vi "Data.vi"(8 "error in (no error)":errorcluster, 11 "PB Msg Template in":refnum<class "Msg.lvclass">) -> (0 "error out":errorcluster, 2 "Data":T1, 3 "PB Msg Template out":refnum<class "Msg.lvclass">)   [LabVIEW 2020, in "Event.lvlib" / "Msg.lvclass"]
uses:
  Msg.lvclass
  Data.ctl
  EventLevel/Enumeration.ctl
  Error/Data.ctl
  Msg.lvclass/Msg.ctl
  Event.lvlib
  Error/Error.lvlib
  EventLevel/EventLevel.lvlib
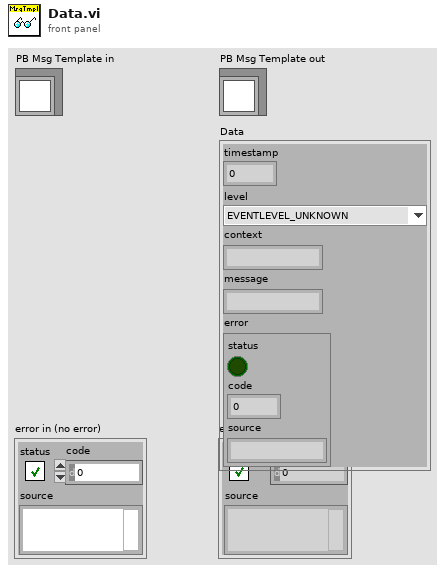
[diagram p1: front panel]
types:
  T1 = typedef "Event.lvlib/Data.ctl" = cluster{"timestamp":i64, "level":T2, "context":string, "message":string, "error":T3}
  T2 = typedef "EventLevel.lvlib/Enumeration.ctl" = enum16{"EVENTLEVEL_UNKNOWN", "EVENTLEVEL_DEBUG", "EVENTLEVEL_INFO", "EVENTLEVEL_WARNING", "EVENTLEVEL_ERROR"}
  T3 = typedef "Error.lvlib/Data.ctl" = errorcluster
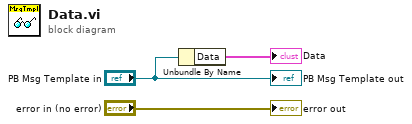
[diagram p0: block diagram]
diagram:
  n1 = Unbundle By Name("PB Msg Template in") -> ("Data"=→"Data":T1)
  "error out" <- "error in (no error)"
  "PB Msg Template out" <- "PB Msg Template in"
